vi "INI Read write path.vi"(5 "key":string, 7 "section":string, 8 "error in":errorcluster, 9 "Default":path, 10 "Path in":path, 11 "Read|Write":T1) -> (0 "error out":errorcluster, 2 "Path out":path)   [LabVIEW 2013]
doc: "This .vi reads/writes a string to the config file. During Write, \"string in\" is passed to \"string out\""
uses:
  Read write mode.ctl
  <vilib>/Utility/config.llb/Read Key (Path).vi
  <vilib>/Utility/config.llb/Write Key (Path).vi
  <vilib>/Utility/config.llb/NI_LVConfig.lvlib
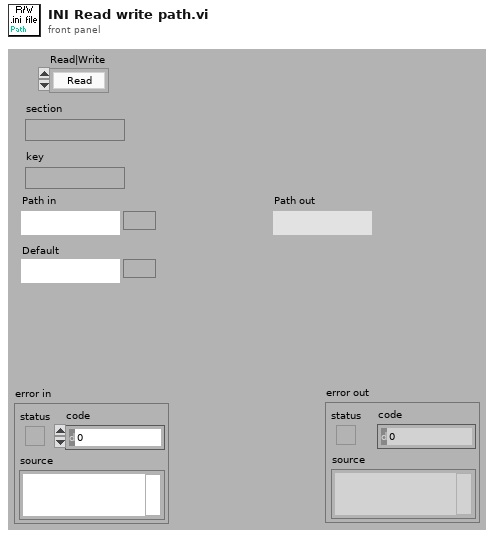
[diagram p1: front panel]
types:
  T1 = typedef "Read write mode.ctl" = enum16{"Read", "Write"}
  T2 = typedef "Semaphore RefNum" = refnum<k1>
  T3 = typedef "NI_LVConfig.lvlib/Config Data RefNum.ctl" = refnum<k1>
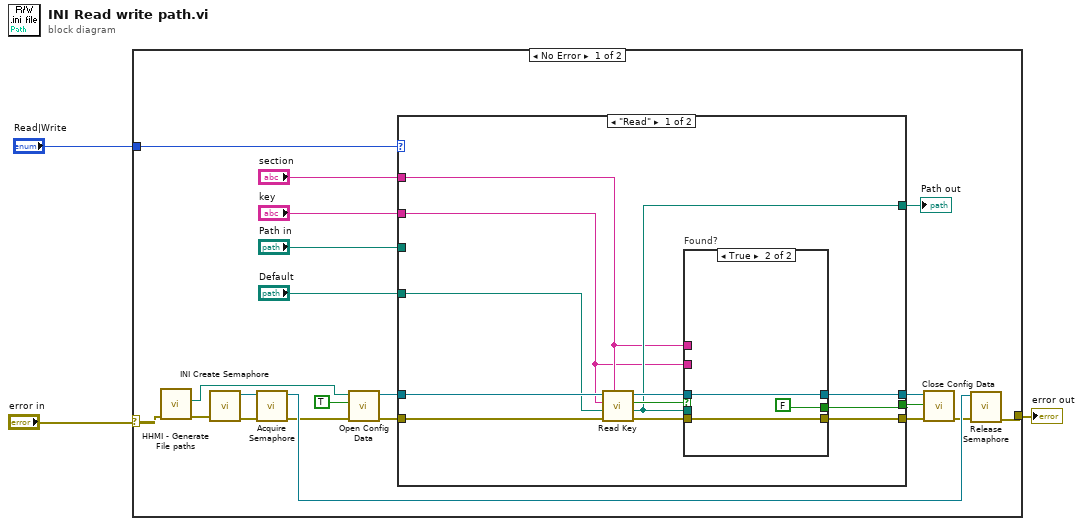
[diagram p0: block diagram]
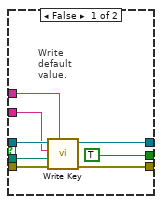
[diagram p2: hidden frame]
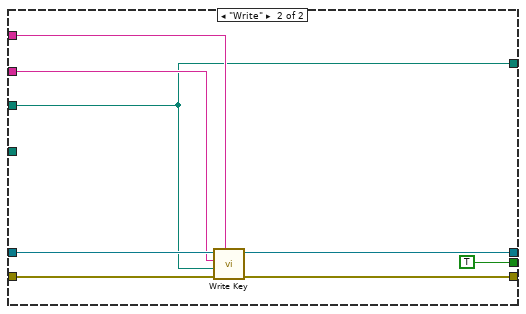
[diagram p3: hidden frame]
diagram:
  n1 = case shown="No Error" "error in" {
    selector: "error in" -> [w6 w56]
    tunnel: "Read|Write" -> [w24 _]
    tunnel: [w9 w56] -> w1
    frame No Error {
      n2 = call "HHMI - Generate File paths.vi"("error in"=w6) -> ("error out"=w5:errorcluster, ".ini path"=w4:path)  [unwired: 8 in, 1 out]
      n3 = call "INI Create Semaphore.vi"("error in"=w5) -> ("error out"=w8:errorcluster, "semaphore"=w7:T2)  [unwired: 1 in, 4 out]
      n4 = call <vilib>:"Acquire Semaphore.vi"("error in (no error)"=w8, "semaphore"=w7) -> ("error out"=w11:errorcluster, "semaphore out"=w12:T2)  [unwired: 1 in, 3 out]
      n5 = call <vilib>:"Open Config Data.vi"("error in (no error)"=w11, "create file if necessary (T)"=TRUE ("create file if necessary? (T)"), "configuration file path"=w4) -> ("error out"=w19:errorcluster, "refnum"=w22:T3)  [unwired: 6 in, 1 out]
      n6 = case shown="\"Read\"" w24 {
        tunnel: [w27 w54] -> w21
        tunnel: w22 -> [w36 w55]
        tunnel: [w26 w53] -> w20
        tunnel: w19 -> [w35 w52]
        tunnel: "section" -> [w29 w51]
        tunnel: "key" -> [w28 w50]
        tunnel: [w30 w48] -> w16
        tunnel: "Path in" -> [_ w48]
        tunnel: [w25 TRUE ("write configuration file? (T)")] -> w14
        tunnel: "Default" -> [w34 _]
        frame "Read" {
          n7 = call-poly <vilib>:"Read Key.vi"("section"=w29, "error in (no error)"=w35, "default value"=w34, "key"=w28, "refnum"=w36) -> ("error out"=w32:errorcluster, "value"=w30:path, "found?"=w33:bool, "refnum out"=w31:T3)  [unwired: 1 in, 2 out]
          n8 = case "Found?" shown="True" w33 {
            tunnel: w32 -> [w44 w47]
            tunnel: [w43 w47] -> w27
            tunnel: w30 -> [w42 _]
            tunnel: w31 -> [w41 w46]
            tunnel: [w40 w46] -> w26
            tunnel: w29 -> [w39 _]
            tunnel: w28 -> [w38 _]
            tunnel: [TRUE ("write configuration file? (T)") FALSE ("write configuration file? (T)")] -> w25
            frame False {
              # "Write\ndefault\nvalue."
              n9 = call-poly <vilib>:"Write Key.vi"("section"=w39, "error in (no error)"=w44, "value"=w42, "key"=w38, "refnum"=w41) -> ("error out"=w43:errorcluster, "refnum out"=w40:T3)  [unwired: 1 in, 4 out]
            }
            frame True {
            }
          }
        }
        frame "Write" {
          n10 = call-poly <vilib>:"Write Key.vi"("section"=w51, "error in (no error)"=w52, "value"=w48, "key"=w50, "refnum"=w55) -> ("error out"=w54:errorcluster, "refnum out"=w53:T3)  [unwired: 1 in, 4 out]
        }
      }
      "Path out" <- w16
      n11 = call <vilib>:"Close Config Data.vi"("error in (no error)"=w21, "write file if changed (T)"=w14, "refnum"=w20) -> ("error out"=w10:errorcluster)  [unwired: 8 out]
      n12 = call <vilib>:"Release Semaphore.vi"("error in (no error)"=w10, "semaphore"=w12) -> ("error out"=w9:errorcluster)  [unwired: 5 out]
    }
    frame Error {
    }
  }
  "error out" <- w1
